vi "example test.vi"() -> ()   [LabVIEW 2013, in "Binary logger tests.lvlib"]
uses:
  Binary logger tests.lvlib
  <vilib>/NI/Tag Bus/tag/Data Type.ctl
  <vilib>/NI/Tag Bus Module Framework/channel/channel classification.ctl
  configuration/Binary datalogger configuration.lvclass
  execution/Binary datalogger runtime.lvclass
  <vilib>/Utility/sysdir.llb/System Directory Type.ctl
  configuration/Binary datalogger configuration.lvclass/Binary datalogger configuration.ctl
  <vilib>/NI/Tag Bus/dictionary/data dictionary.lvclass/data dictionary.ctl
  <vilib>/NI/Tag Bus/dictionary/lookup polymorphs/locate double.vi
  <vilib>/NI/Tag Bus/table/data polymorphs/write one/write Double.vi
  configuration/Write channels.vi
  configuration/Write backup directory.vi
  configuration/Write Path.vi
  <vilib>/NI/Tag Bus/dictionary/search/find data index.vi
  <vilib>/NI/Tag Bus/dictionary/search/search string list.vi
  <vilib>/NI/Tag Bus/dictionary/tag not found.vi
  <vilib>/NI/Tag Bus Module Framework/channel/TBM channel.lvclass
  <vilib>/NI/Tag Bus/tag/tag descriptor.lvclass
  <vilib>/NI/Tag Bus/dictionary/data dictionary.lvclass
  <vilib>/NI/Tag Bus/table/data table.lvlib
  <vilib>/NI/Configuration Framework/serializable configuration/NISE_CEF_serializable configuration.lvclass
panel:
  out "final error":errorcluster
  out "output error":errorcluster
  out "output lookup error":errorcluster
  out "init error":errorcluster
  out "correct execution settings":bool
  out "serialization problem":errorcluster
  out "invalid configuration":errorcluster
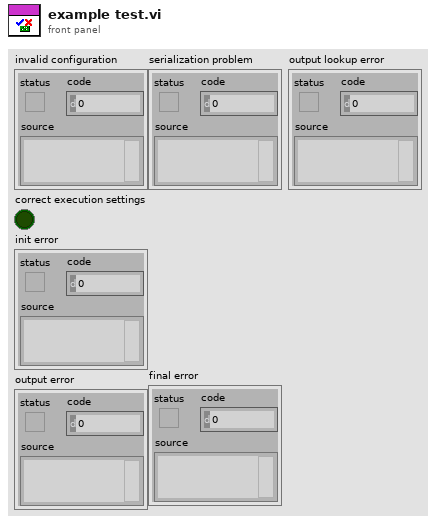
[diagram p1: front panel]
types:
  T1 = typedef "System Directory Type.ctl" = i32
  T2 = typedef "TBM channel.lvclass/channel classification.ctl" = enum16{"input data", "output data", "processing parameter", "processing result"}
  T3 = typedef "tag bus.lvlib/tag descriptor.lvclass/Data Type.ctl" = enum16{"Double", "Single", "I64", "I32", "I16", "I8", "U64", "U32", "U16", "U8", "Boolean", "String", "Array of Double", "Array of Single", "Array of I64", "Array of I32", "Array of I16", "Array of I8", "Array of U64", "Array of U32", "Array of U16", "Array of U8", "Array of Boolean", "Array of String"}
  T4 = typedef "TBM channel.lvclass/data tables.ctl" = cluster{"input data":T5, "processing parameter":T5, "processing result":T5, "output data":T5}
  T5 = typedef "tag bus.lvlib/dictionary table pair.ctl" = cluster{"data dictionary":refnum<class "data dictionary.lvclass">, "data table":T6}
  T6 = typedef "tag bus.lvlib/data table.lvlib/data table.ctl" = cluster{"Double":dbl[], "Single":sgl[], "I64":i64[], "I32":i32[], "I16":i16[], "I8":i8[], "U64":u64[], "U32":u32[], "U16":u16[], "U8":u8[], "Boolean":bool[], "String":string[], "Array of Double":cluster{"DBL Array":dbl[]}[], "Array of Single":cluster{"SGL Array":sgl[]}[], "Array of I64":cluster{"I64 Array":i64[]}[], "Array of I32":cluster{"I32 Array":i32[]}[], "Array of I16":cluster{"I16 Array":i16[]}[], "Array of I8":cluster{"I8 Array":i8[]}[], "Array of U64":cluster{"U64 Array":u64[]}[], "Array of U32":cluster{"U32 Array":u32[]}[], "Array of U16":cluster{"U16 Array":u16[]}[], "Array of U8":cluster{"U8 Array":u8[]}[], "Array of Boolean":cluster{"Boolean Array":bool[]}[], "Array of String":cluster{"String Array":string[]}[]}
  T7 = typedef "TBM module execution interface.lvclass/execution settings.ctl" = cluster{"reads inputs":bool, "processes data":bool, "writes outputs":bool}
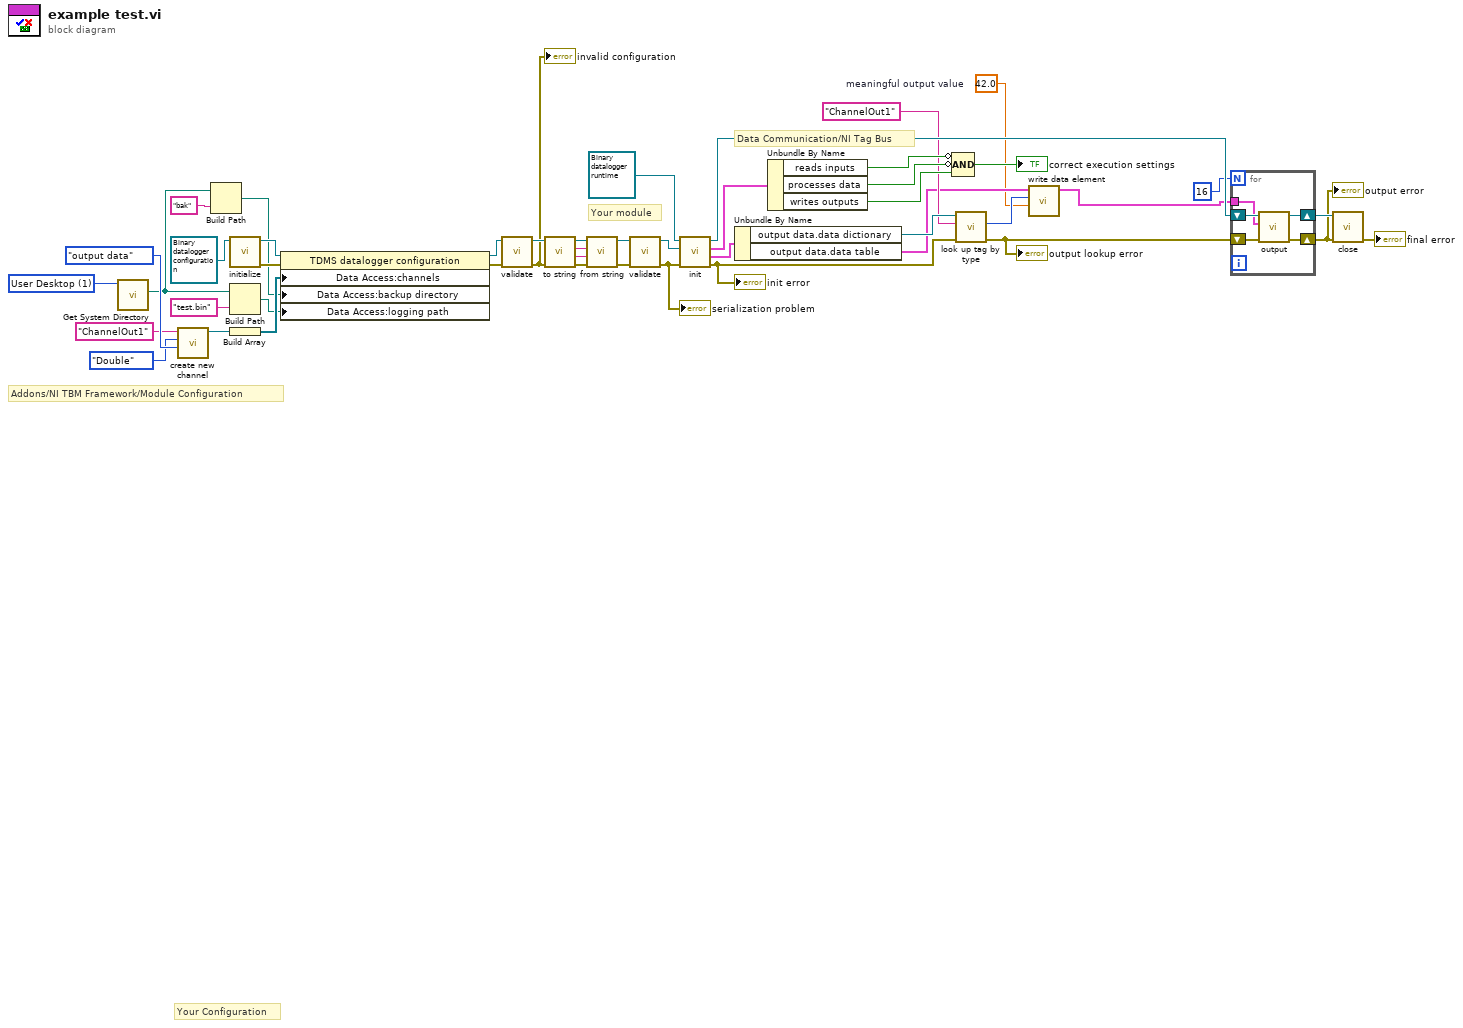
[diagram p0: block diagram]
diagram:
  w7 = T1 1 items=["User Home"=0, "User Desktop"=1, "User Documents"=2, "User Application Data"=3, "User Preferences"=4, "User Temporary"=5, "Public Documents"=6, "Public Application Data"=7, "Public Preferences"=8, "Public Cache"=13, "System Core Libraries"=9, "System Installed Libraries"=10, "Application Files"=11, "Boot Volume Root"=12] ("system directory type")
  w21 = 42.0  # meaningful output value
  # "Data Communication/NI Tag Bus"
  # "Your module"
  # "Your Configuration"
  # "Addons/NI TBM Framework/Module Configuration"
  n1 = call <vilib>:"Get System Directory.vi"("system directory type"=w7) -> ("system directory"=w3:path)  [unwired: 10 in]
  n2 = call <vilib>:"create new channel.vi"("channel classification"=channel_classification."output data", "data type"=Data_Type."Double", "channel name"="ChannelOut1") -> ("channel"=w15:refnum<class "TBM channel.lvclass">)  [unwired: 8 in]
  n3 = Build Path(base path=w3, name or relative path="bak") -> (appended path=w5:path)
  n4 = call <vilib>:"initialize.vi"("configuration in"=refnum<class "Binary datalogger configuration.lvclass"> refnum ("TDMS datalogger configuration")) -> ("error out"=w8:errorcluster, "configuration out"=w9:refnum<class "Binary datalogger configuration.lvclass">)  [unwired: 8 in, 1 out]
  n5 = Build Path(base path=w3, name or relative path="test.bin") -> (appended path=w2:path)
  n6 = Build Array(w15) -> (w12:refnum<class "TBM channel.lvclass">[])
  n7 = property class="TDMS datalogger configuration"(reference=w9, error in=w8, "Data Access:channels"=w12, "Data Access:backup directory"=w5, "Data Access:logging path"=w2) -> (reference out=w14:refnum<class "Binary datalogger configuration.lvclass">, error out=w13:errorcluster)
  n8 = call-dynamic "validate.vi"("error in"=w13, "bin datalogger configuration in"=w14) -> ("error out"=w42:errorcluster, "bin datalogger configuration out"=w43:refnum<class "Binary datalogger configuration.lvclass">)  [unwired: 8 in]
  "invalid configuration" <- w42
  n9 = call-dynamic "to string.vi"("error in"=w42, "bin datalogger configuration in"=w43) -> ("error out"=w38:errorcluster, "data"=w39:string, "version"=w40:string, "bin datalogger configuration out"=w41:refnum<class "Binary datalogger configuration.lvclass">)  [unwired: 6 in]
  n10 = call-dynamic "from string.vi"("error in"=w38, "data"=w39, "version"=w40, "bin datalogger configuration in"=w41) -> ("error out"=w36:errorcluster, "bin datalogger configuration out"=w37:refnum<class "Binary datalogger configuration.lvclass">)  [unwired: 6 in]
  n11 = call-dynamic "validate.vi"("error in"=w36, "bin datalogger configuration in"=w37) -> ("error out"=w35:errorcluster, "bin datalogger configuration out"=w34:refnum<class "Binary datalogger configuration.lvclass">)  [unwired: 8 in]
  "serialization problem" <- w35
  n12 = call-dynamic "init.vi"("error in"=w35, "TBM module configuration in"=w34, "bin datalogger runtime in"=refnum<class "Binary datalogger runtime.lvclass"> refnum ("TDMS datalogger runtime")) -> ("error out"=w27:errorcluster, "data allocations"=w28:T4, "execution settings"=w33:T7, "bin datalogger runtime out"=w26:refnum<class "Binary datalogger runtime.lvclass">)  [unwired: 5 in]
  "init error" <- w27
  n13 = Unbundle By Name(w28) -> ("output data.data dictionary"=w25:refnum<class "data dictionary.lvclass">, "output data.data table"=w22:T6)
  n14 = Unbundle By Name(w33) -> ("reads inputs"=w30:bool, "processes data"=w32:bool, "writes outputs"=w31:bool)
  n15 = Compound Arithmetic op=AND(invert w30, invert w32, w31) -> (→"correct execution settings":bool)
  n16 = call-poly <vilib>:"look up tag by type.vi"("error in"=w27, "name"="ChannelOut1" ("channel name"), "data dictionary in"=w25) -> ("error out"=w20:errorcluster, "index"=w23:i32)  [unwired: 6 in, 1 out]
  "output lookup error" <- w20
  n17 = call-poly <vilib>:"write data element.vi"("value"=w21, "index"=w23, "data table in"=w22) -> ("data table out"=w19:T6)  [unwired: 8 in]
  n18 = for {
    N: 16 -> [_]
    tunnel: w19 -> [w49]
    shift-right: [w48] -> w18
    shift-left: w26 -> [w51]
    shift-right: [w47] -> w17
    shift-left: w20 -> [w50]
    n19 = call-dynamic "output.vi"("error in"=w50, "data table in"=w49, "bin datalogger runtime in"=w51) -> ("error out"=w47:errorcluster, "bin datalogger runtime out"=w48:refnum<class "Binary datalogger runtime.lvclass">)  [unwired: 6 in, 1 out]
  }
  "output error" <- w17
  n20 = call-dynamic "close.vi"("error in"=w17, "bin datalogger runtime in"=w18) -> ("error out"=→"final error":errorcluster)  [unwired: 9 in]
